vi "StackLocation.vi"(11 "Mode":T1(ring)=enum."Retrieve Stack Location") -> (2 "Current\nWindDirection":dbl, 3 "StackPosition (at 0deg)":sgl[](array[numeric]))   [LabVIEW 2015]
uses:
  ADAM Client/Sub VIs/ADAM Controls/Update_scan_value.ctl
  Trav_mode.ctl
  Controls/User_Specific_mode.ctl
  Globals/Preference_global.vi
  Globals/Trav_pos_global.vi
panel:
  in  "Extra Command String":string
  out "MeasuredStackPosition":sgl[](array[numeric]) format="%.2f"
  # "• First, check the probe is correctly zeroed at TT centre.\n• Next, position the probe directly over the stack under study, with the turntable at any angle you like.\n• Then select \"Record Stack Location\" mode, and run this VI."
  # "@"
  # "="
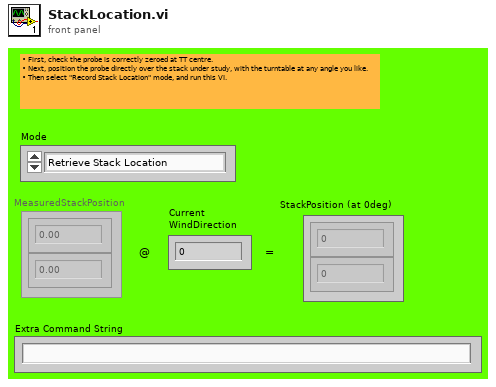
[diagram p1: front panel]
types:
  T1 = enum16{"Record Stack Location", "Retrieve Stack Location"}
  T2 = enum8{"Enabled", "Disabled", "Disabled and Grayed Out"}
  T3 = typedef "User_Specific_mode.ctl" = enum16{"Check VI only", "Run VI"}
  T4 = typedef "Trav_mode.ctl" = enum16{"Move traverse", "Read traverse position", "Teach Position"}
  T5 = typedef "Update_scan_value.ctl" = cluster{"Channel Name":string, "New Value":dbl}
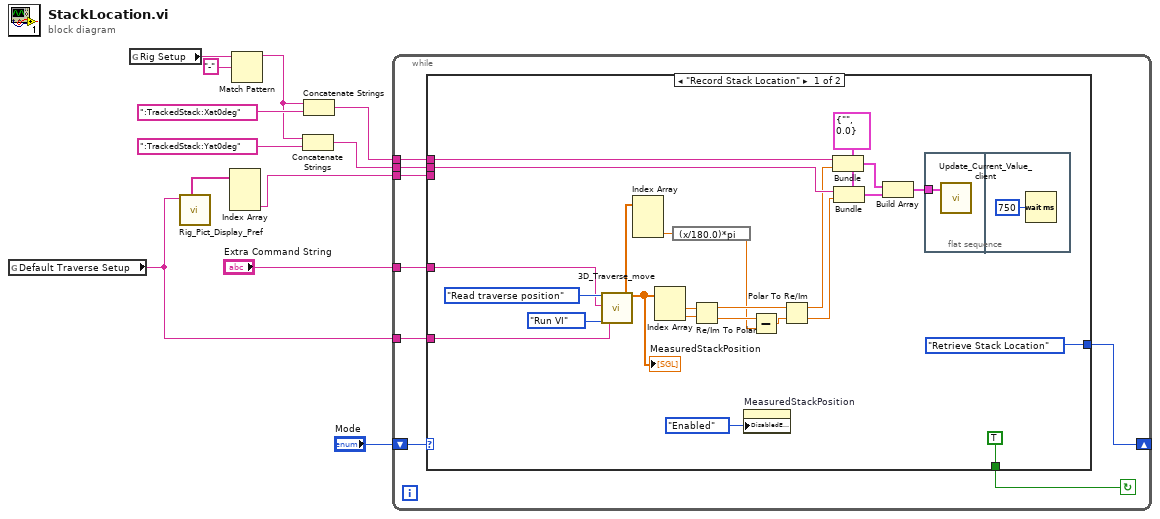
[diagram p0: block diagram]
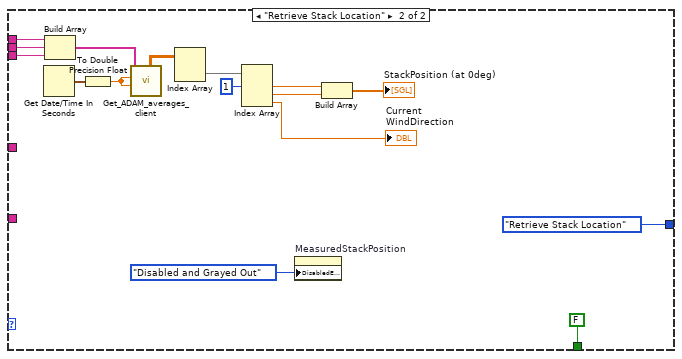
[diagram p2: hidden frame]
diagram:
  n1 = global read "Trav_pos_global.vi" "Default Traverse Setup"() -> (w4:string)
  n2 = global read "Preference_global.vi" "Rig Setup"() -> (w9:string)
  n3 = call "Rig_Pict_Display_Pref.vi"("Traverse Name"=w4) -> ("Roll Pitch Yaw ADAM Channels"=w3:string[])  [unwired: 3 in, 4 out]
  n4 = Index Array(array=w3) -> (element #3=w2:string)  [unwired: 3 in, 2 out]
  n5 = Match Pattern(string=w9, regular expression="-") -> (before substring=w8:string)  [unwired: 4 out]
  n6 = Concatenate Strings(w8, ":TrackedStack:Yat0deg") -> (w6:string)
  n7 = Concatenate Strings(w8, ":TrackedStack:Xat0deg") -> (w5:string)
  n8 = while {
    shift-right: [w18] -> _
    shift-left: "Mode" -> [w20]
    tunnel: w2 -> [w17]
    tunnel: w6 -> [w16]
    tunnel: w5 -> [w15]
    tunnel: w4 -> [w14]
    tunnel: "Extra Command String" -> [w13]
    stop <- w19 continue-if-true
    n9 = case shown="\"Record Stack Location\"" w20 {
      tunnel: [TRUE FALSE] -> w19
      tunnel: [T1."Retrieve Stack Location" ("Mode") T1."Retrieve Stack Location" ("Mode")] -> w18
      tunnel: w17 -> [_ w50]
      tunnel: w16 -> [w40 w49]
      tunnel: w15 -> [w41 w48]
      tunnel: w14 -> [w23 _]
      tunnel: w13 -> [w21 _]
      frame "Record Stack Location" {
        w42 = T5 {"Channel Name"="", "New Value"=0.0} ("Update Scan Value Cluster")
        n10 = call "3D_Traverse_move.vi"("Mode"=Trav_mode."Read traverse position", "Extra command String"=w21, "Simulate/Run"=User_Specific_mode."Run VI", "Traverse name"=w23) -> ("Model:    Roll        Pitch         Yaw  (deg)"=w25:sgl[], "Trav Position achieved"=w34:sgl[])  [unwired: 13 in, 1 out]
        "MeasuredStackPosition" <- w34
        n11 = Index Array(array=w25) -> (element #3=w24:sgl)  [unwired: 3 in, 2 out]
        n12 = Index Array(array=w34) -> (element #1=w29:sgl, element #2=w28:sgl)  [unwired: 2 in]
        n13 = expression code="(x/180.0)*pi" ("degrees to radians")(w24) -> (w30:sgl)
        n14 = Re/Im To Polar(2:w28, 3:w29) -> (0:w32:sgl, 1:w33:sgl)
        n15 = property on="MeasuredStackPosition" class="Arr (strict)"("DisabledEnum"=T2."Enabled" ("Disabled")) -> ()  [unwired: 2 in, 2 out]
        n16 = Subtract(x=w32, y=w30) -> (x-y=w31:sgl)
        n17 = Polar To Re/Im(2:w31, 3:w33) -> (0:w26:sgl, 1:w27:sgl)
        n18 = Bundle(cluster=w42, "Channel Name"=w41, "New Value"=w27) -> (w38:T5)
        n19 = Bundle(cluster=w42, "Channel Name"=w40, "New Value"=w26) -> (w39:T5)
        n20 = Build Array(w38, w39) -> (w37:T5[])
        n21 = flat-sequence {
          tunnel: w37 -> [w45]
          frame #0 {
            n22 = call "Update_Current_Value_client.vi"("Update array in"=w45) -> ()  [unwired: 1 in]
          }
          frame #1 {
            n23 = Wait (ms)(milliseconds to wait=u32 750) -> ()  [unwired: 1 out]
          }
        }
      }
      frame "Retrieve Stack Location" {
        n24 = Get Date/Time In Seconds() -> (seconds since 1Jan1904=w60:timestamp)
        n25 = Build Array(w48, w49, w50) -> (w51:string[])
        n26 = To Double Precision Float(number=w60) -> (double precision float=w59:dbl)
        n27 = call "Get_ADAM_averages_client.vi"("End time"=w59, "Start time"=w59, "ADAM Ch Names"=w51) -> ("DBL values"=w58:dbl[][])  [unwired: 2 in, 6 out]
        n28 = Index Array(array=w58) -> (element=w57:dbl[])  [unwired: 2 in]
        n29 = Index Array(array=w57, index #1=1 ("index")) -> (element #1=w55:dbl, element #2=w54:dbl, element #3=→"Current\nWindDirection":dbl)  [unwired: 2 in]
        n30 = property on="MeasuredStackPosition" class="Arr (strict)"("DisabledEnum"=T2."Disabled and Grayed Out" ("Disabled")) -> ()  [unwired: 2 in, 2 out]
        n31 = Build Array(w55, w54) -> (→"StackPosition (at 0deg)":dbl[])
      }
    }
  }
